vi "Read Configurations.vi"(0 "Hotel Management Tool Model in":refnum<class "Hotel Management Tool Model.lvclass">, 11 "error in (no error)":errorcluster) -> (4 "Hotel Management Tool Model out":refnum<class "Hotel Management Tool Model.lvclass">, 15 "error out":errorcluster)   [LabVIEW 2023, in "Hotel Management Tool Model.lvlib" / "Hotel Management Tool Model.lvclass"]
uses:
  Hotel Management Tool Model.lvclass
  Hotel Management Tool Model.lvclass/Hotel Management Tool Model.ctl
  <vilib>/Utility/config.llb/Read Key (Boolean).vi
  Utilities/Utilities.lvlib
  <vilib>/Utility/config.llb/NI_LVConfig.lvlib
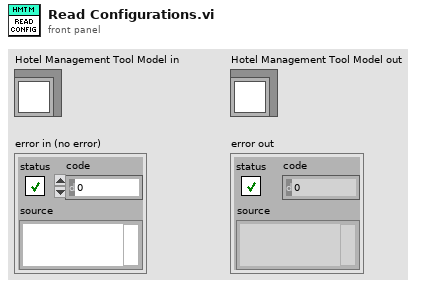
[diagram p1: front panel]
types:
  T1 = typedef "NI_LVConfig.lvlib/Config Data RefNum.ctl" = refnum<k1>
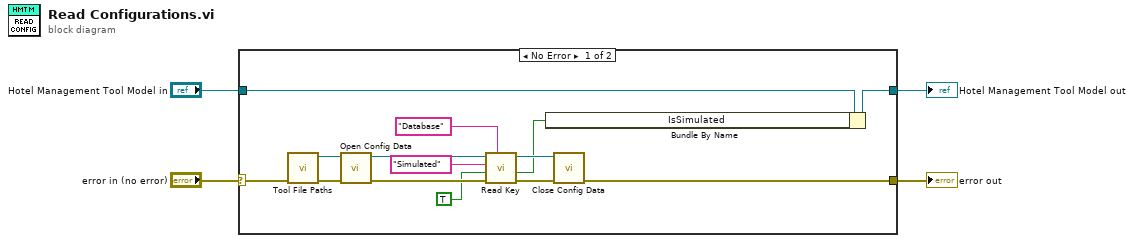
[diagram p0: block diagram]
diagram:
  n1 = case shown="No Error" "error in (no error)" {
    selector: "error in (no error)" -> [w18 w19]
    tunnel: "Hotel Management Tool Model in" -> [w17 w20]
    tunnel: [w16 w20] -> w2
    tunnel: [w10 w19] -> w1
    frame No Error {
      n2 = call "Tool File Paths.vi"("error in (no error)"=w18) -> ("Tool Configuration File Path"=w9:path, "error out"=w11:errorcluster)  [unwired: 12 in, 1 out]
      n3 = call <vilib>:"Open Config Data.vi"("error in (no error)"=w11, "configuration file path"=w9) -> ("error out"=w14:errorcluster, "refnum"=w15:T1)  [unwired: 7 in, 1 out]
      n4 = call-poly <vilib>:"Read Key.vi"("section"="Database", "error in (no error)"=w14, "default value"=TRUE, "key"="Simulated", "refnum"=w15) -> ("error out"=w12:errorcluster, "value"=w6:bool, "refnum out"=w13:T1)  [unwired: 3 in, 1 out]
      n5 = Bundle By Name(cluster=w17, "IsSimulated"=w6) -> (w16:refnum<class "Hotel Management Tool Model.lvclass">)
      n6 = call <vilib>:"Close Config Data.vi"("error in (no error)"=w12, "refnum"=w13) -> ("error out"=w10:errorcluster)  [unwired: 8 in, 1 out]
    }
    frame Error {
    }
  }
  "error out" <- w1
  "Hotel Management Tool Model out" <- w2
